vi "Broken Test 0001.vi"(8 "error in (no error)":errorcluster) -> (0 "error out":errorcluster)   [LabVIEW 2013]
uses:
  classes/Assert/Assert.lvclass
  classes/Test/Test.lvclass
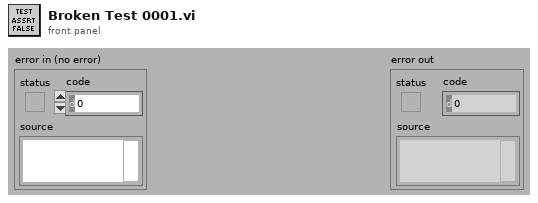
[diagram p1: front panel]
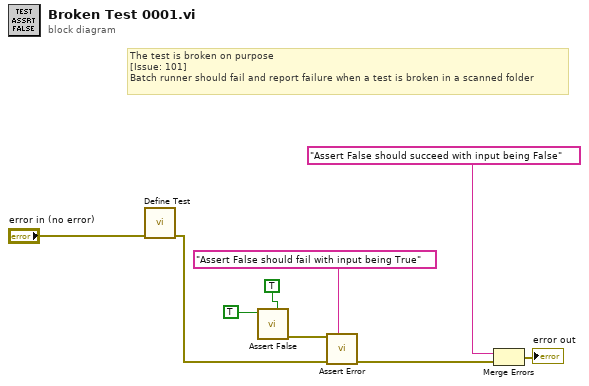
[diagram p0: block diagram]
diagram:
  # "The test is broken on purpose\n[Issue: 101]\nBatch runner should fail and report failure when a test is broken in a scanned folder"
  n1 = call "Define Test.vi"("error in (no error)"="error in (no error)") -> ("error out"=w2:errorcluster)  [unwired: 10 in]
  n2 = call "Assert False.vi"("Assert Only? (F)"=TRUE, "False?"=TRUE ("True?")) -> ("error out"=w8:errorcluster)  [unwired: 9 in]
  n3 = call "Assert Error.vi"("Label"="Assert False should fail with input being True", "error in (no error)"=w2, "Error?"=w8) -> ("error out"=w4:errorcluster)  [unwired: 8 in]
  n4 = Merge Errors("Assert False should succeed with input being False" ("Label"), w4) -> (→"error out":errorcluster)
